vi "AVARVAREI_7SEGMENT.vi"(1 "INPUT":T1, 2 "SELECTIA CIFRA":string) -> (0 "OUTPUT":T1)   [LabVIEW 2025]
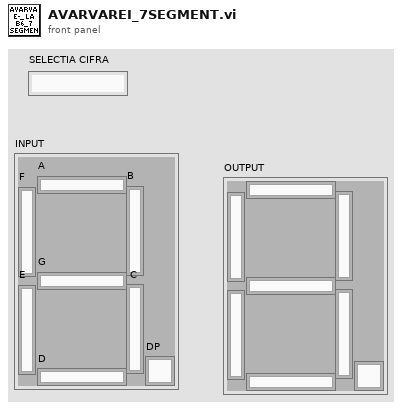
[diagram p1: front panel]
types:
  T1 = cluster{"A":bool, "G":bool, "D":bool, "B":bool, " C":bool, "F":bool, "E":bool, "DP":bool}
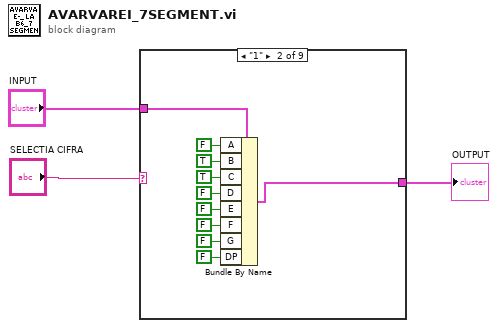
[diagram p0: block diagram]
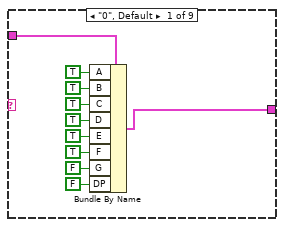
[diagram p2: hidden frame]
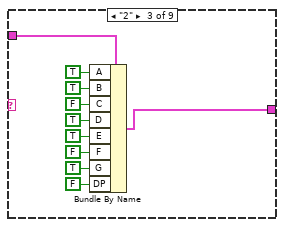
[diagram p3: hidden frame]
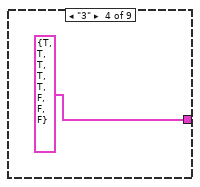
[diagram p4: hidden frame]
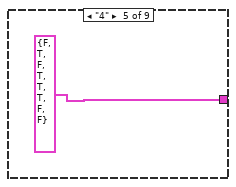
[diagram p5: hidden frame]
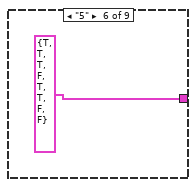
[diagram p6: hidden frame]
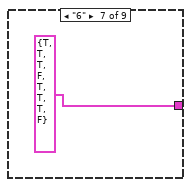
[diagram p7: hidden frame]
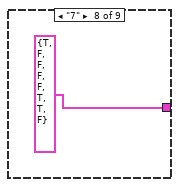
[diagram p8: hidden frame]
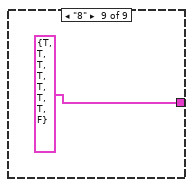
[diagram p9: hidden frame]
diagram:
  n1 = case shown="\"1\"" "SELECTIA CIFRA" {
    tunnel: "INPUT" -> [w13 w23 w33 _ _ _ _ _ _]
    tunnel: [w12 w22 w32 T1 {"A"=TRUE, "G"=TRUE, "D"=TRUE, "B"=TRUE, " C"=TRUE, "F"=FALSE, "E"=FALSE, "DP"=FALSE} ("INPUT") T1 {"A"=FALSE, "G"=TRUE, "D"=FALSE, "B"=TRUE, " C"=TRUE, "F"=TRUE, "E"=FALSE, "DP"=FALSE} ("INPUT") T1 {"A"=TRUE, "G"=TRUE, "D"=TRUE, "B"=FALSE, " C"=TRUE, "F"=TRUE, "E"=FALSE, "DP"=FALSE} ("INPUT") T1 {"A"=TRUE, "G"=TRUE, "D"=TRUE, "B"=FALSE, " C"=TRUE, "F"=TRUE, "E"=TRUE, "DP"=FALSE} ("INPUT") T1 {"A"=TRUE, "G"=FALSE, "D"=FALSE, "B"=FALSE, " C"=FALSE, "F"=TRUE, "E"=TRUE, "DP"=FALSE} ("INPUT") T1 {"A"=TRUE, "G"=TRUE, "D"=TRUE, "B"=TRUE, " C"=TRUE, "F"=TRUE, "E"=TRUE, "DP"=FALSE} ("INPUT")] -> w1
    frame "0", Default {
      n2 = Bundle By Name "Bundle By Name"(cluster=w13, "A"=TRUE, "B"=TRUE, "C"=TRUE, "D"=TRUE, "E"=TRUE, "F"=TRUE, "G"=FALSE, "DP"=FALSE) -> (w12:T1)
    }
    frame "1" {
      n3 = Bundle By Name "Bundle By Name"(cluster=w23, "A"=FALSE, "B"=TRUE, "C"=TRUE, "D"=FALSE, "E"=FALSE, "F"=FALSE, "G"=FALSE, "DP"=FALSE) -> (w22:T1)
    }
    frame "2" {
      n4 = Bundle By Name "Bundle By Name"(cluster=w33, "A"=TRUE, "B"=TRUE, "C"=FALSE, "D"=TRUE, "E"=TRUE, "F"=FALSE, "G"=TRUE, "DP"=FALSE) -> (w32:T1)
    }
    frame "3" {
    }
    frame "4" {
    }
    frame "5" {
    }
    frame "6" {
    }
    frame "7" {
    }
    frame "8" {
    }
  }
  "OUTPUT" <- w1
